vi "Read Header.vi"(11 "CSV File Sink in":refnum<class "CSV File Sink.lvclass">) -> (2 "Header":string, 3 "CSV File Sink out":refnum<class "CSV File Sink.lvclass">)   [LabVIEW 2016, in "Stream Log.lvlib" / "CSV File Sink.lvclass"]
uses:
  <userlib>/Composed Systems/Stream/Log/CSV File Sink/CSV File Sink.lvclass
  <userlib>/Composed Systems/Stream/Log/CSV File Sink/CSV File Sink.lvclass/CSV File Sink.ctl
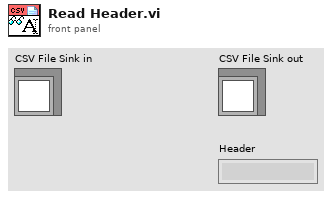
[diagram p1: front panel]
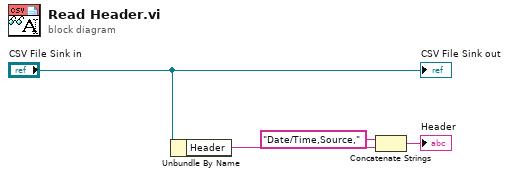
[diagram p0: block diagram]
diagram:
  n1 = Unbundle By Name("CSV File Sink in") -> ("Header"=w3:string)
  n2 = Concatenate Strings("Date/Time,Source," ("string"), w3) -> (→"Header":string)
  "CSV File Sink out" <- "CSV File Sink in"
